vi "BRig_dataLC_Wrong_nRew2_l1.vi"() -> (2 "output_Wrong_nRew2_l1":i32)   [LabVIEW 2014]
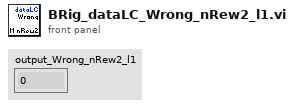
[diagram p1: front panel]
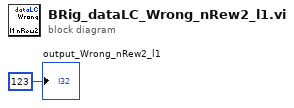
[diagram p0: block diagram]
diagram:
  "output_Wrong_nRew2_l1" <- 123 ("output_iBlock")
